vi "PicohrdlReady.vi"(8 "error in (no error)":errorcluster, 11 "handle in":i16) -> (0 "error out":errorcluster, 3 "handle out":i16, 6 "ready":i16)   [LabVIEW 2010]
doc: "Calls IsReady() to check if data is ready from unit."
uses:
  PicoHRDL.dll
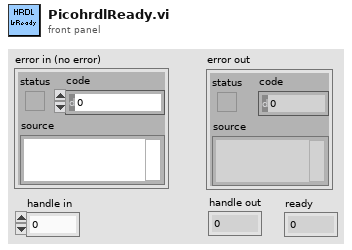
[diagram p1: front panel]
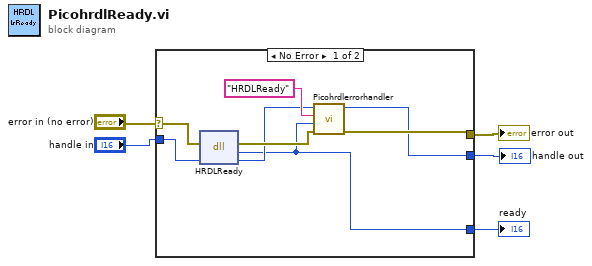
[diagram p0: block diagram]
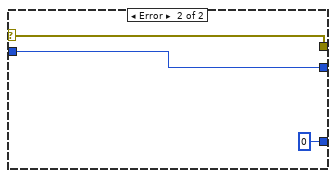
[diagram p2: hidden frame]
diagram:
  n1 = case shown="No Error" "error in (no error)" {
    selector: "error in (no error)" -> [w13 w15]
    tunnel: "handle in" -> [w12 w16]
    tunnel: [w7 w16] -> w5
    tunnel: [w10 w15] -> w4
    tunnel: [w6 i16 0 ("ready")] -> w3
    frame No Error {
      n2 = dll-call lib="PicoHRDL.dll" fn="HRDLReady"(error in=w13, "handle"=w12) -> (error out=w11:errorcluster, "ready"=w6:i16, "handle"=w8:i16)  [unwired: 2 in, 1 out]
      n3 = call "Picohrdlerrorhandler.vi"("Handle in"=w8, "API function"="HRDLReady", "Return"=w6, "error in (no error)"=w11) -> ("Handle out"=w7:i16, "error out"=w10:errorcluster)  [unwired: 5 in]
    }
    frame Error {
    }
  }
  "error out" <- w4
  "handle out" <- w5
  "ready" <- w3
